vi "LIDAR-Test-On-cRIO.vi"() -> ()   [LabVIEW 2010]
uses:
  3.2.1-LIDAR Data Typedef.ctl
  <instrlib>/Hokuyo URG Series/Public/Initialize-Standard.vi
  3.0-Global.vi
  <instrlib>/Hokuyo URG Series/Hokuyo URG Series.lvlib
panel:
  out "Angle Array":dbl[](array[numeric])
  out "Magnitude Array":dbl[](array[numeric])
  in  "ID Query?":bool
  in  "VISA resource name":refnum<visa-resource-name>="TCPIP::10.10.10.15::10940::Socket"
  in  "Stop":bool
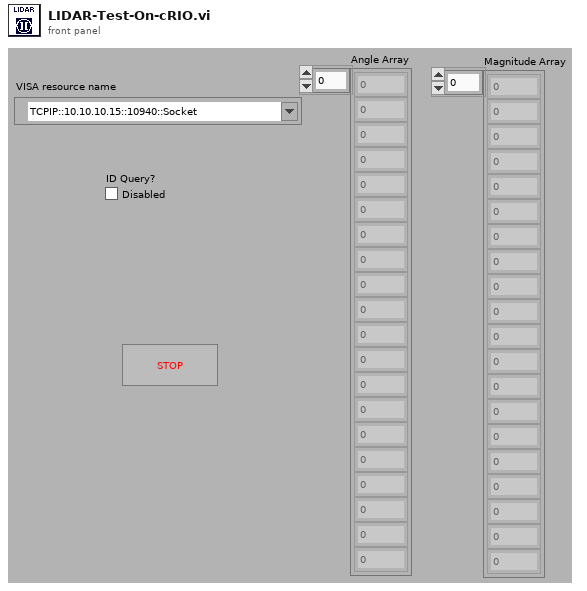
[diagram p1: front panel]
types:
  T1 = typedef "3.2.1-LIDAR Data Typedef.ctl" = cluster{"Angle array":dbl[], "Magnitude array ":dbl[]}
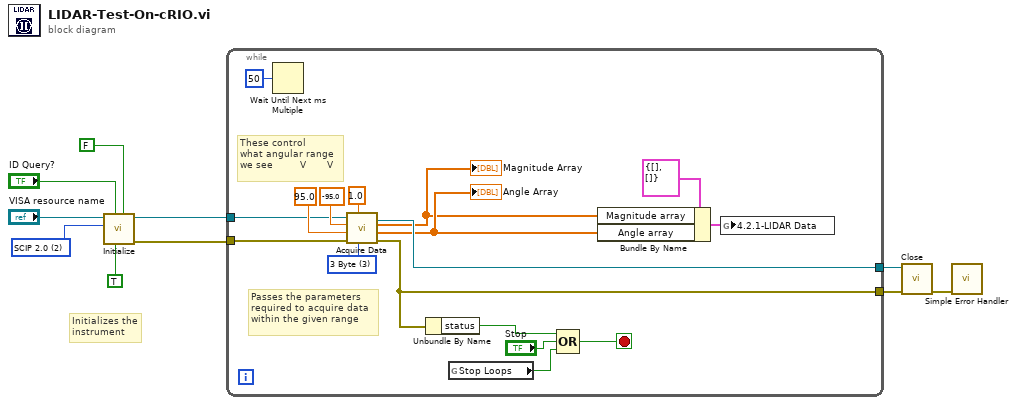
[diagram p0: block diagram]
diagram:
  w1 = u32 2 items=["Convert to Latest", "SCIP 1.1", "SCIP 2.0", "SCIP 2.2"] ("Protocol (2: SCIP 2.0)")
  # "Initializes the instrument"
  n1 = call-poly <instrlib>:"Initialize.vi"("Reset? (F: No)"=FALSE ("Reset Instrument (Disabled)"), "Checksum (Disabled)"=TRUE ("Checksum"), "ID Query? (Enabled)"="ID Query?", "Protocol (2: SCIP 2.0)"=w1, "VISA resource name"="VISA resource name") -> ("error out"=w2:errorcluster, "VISA resource name out"=w3:refnum<visa-resource-name>)  [unwired: 5 in]
  n2 = while {
    tunnel: w3 -> [w21]
    tunnel: [w17] -> w10
    tunnel: [w18] -> w4
    tunnel: w2 -> [w20]
    stop <- w25 stop-if-true
    w19 = u16 3 items=["2 Byte"=2, "3 Byte"=3] ("Encoding Width")
    # "These control\nwhat angular range\nwe see         V       V"
    # "Passes the parameters\nrequired to acquire data\nwithin the given range"
    n3 = Wait Until Next ms Multiple(millisecond multiple=u32 50) -> ()  [unwired: 1 out]
    n4 = call <instrlib>:"Acquire Data.vi"("Data Encoding Width (3 Byte)"=w19, "Cluster Count (1)"=1.0 ("Cluster Count"), "error in (no error)"=w20, "End Point (120°)"=95.0 ("End Point"), "Start Point (-120°)"=-95.0 ("Start Point"), "VISA resource name"=w21) -> ("error out"=w17:errorcluster, "Direction"=w15:dbl[], "Magnitude"=w14:dbl[], "VISA resource name out"=w18:refnum<visa-resource-name>)  [unwired: 2 in]
    "Magnitude Array" <- w14
    "Angle Array" <- w15
    n5 = Unbundle By Name(w17) -> ("status"=w27:bool)
    n6 = global read "3.0-Global.vi" "Stop Loops"() -> (w11:bool)
    n7 = Compound Arithmetic op=OR(w27, "Stop", w11) -> (w25:bool)
    n8 = Bundle By Name(cluster=T1 {"Angle array"=[], "Magnitude array "=[]} ("LIDAR Data"), "Magnitude array"=w14, "Angle array"=w15) -> (w12:T1)
    n9 = global write "3.0-Global.vi" "4.2.1-LIDAR Data"(w12) -> ()
  }
  n10 = call <instrlib>:"Close.vi"("error in (no error)"=w10, "VISA resource name"=w4) -> ("error out"=w7:errorcluster)  [unwired: 9 in]
  n11 = call <vilib>:"Simple Error Handler.vi"("error in (no error)"=w7) -> ()  [unwired: 4 in, 5 out]
